vi "_PT_2DMCT_Example.vi"() -> ()   [LabVIEW 2026]
panel:
  out "ExtChData":dbl[][](array[numeric])
  in  "Timeout":i32
  in  "ExChs":i32
  in  "Frames":i32=1
  in  "Acq Trigger?":bool
  in  "Offset":i32=128 min=0 max=255 step=1
  out "Actual (us)":dbl
  in  "IntegrationTime (us)":dbl=0.1 min=0.1 max=5000.0 step=0.1
  out "MaxFrameRate":dbl
  in  "Frame Size (Row x Col)":u16(ring) items=["128x128", "96x128", "64x128", "32x128"]
  out "TempK":dbl
  out "First Image":dbl[][](graph)
  out "error":errorcluster
  # "INPUTS"
  # "OUTPUTS"
  # "Get Temp:"
  # "Set Frame Size:\n(optional)"
  # "Set Integration Time:"
  # "Set Offset:"
  # "Get Frames:"
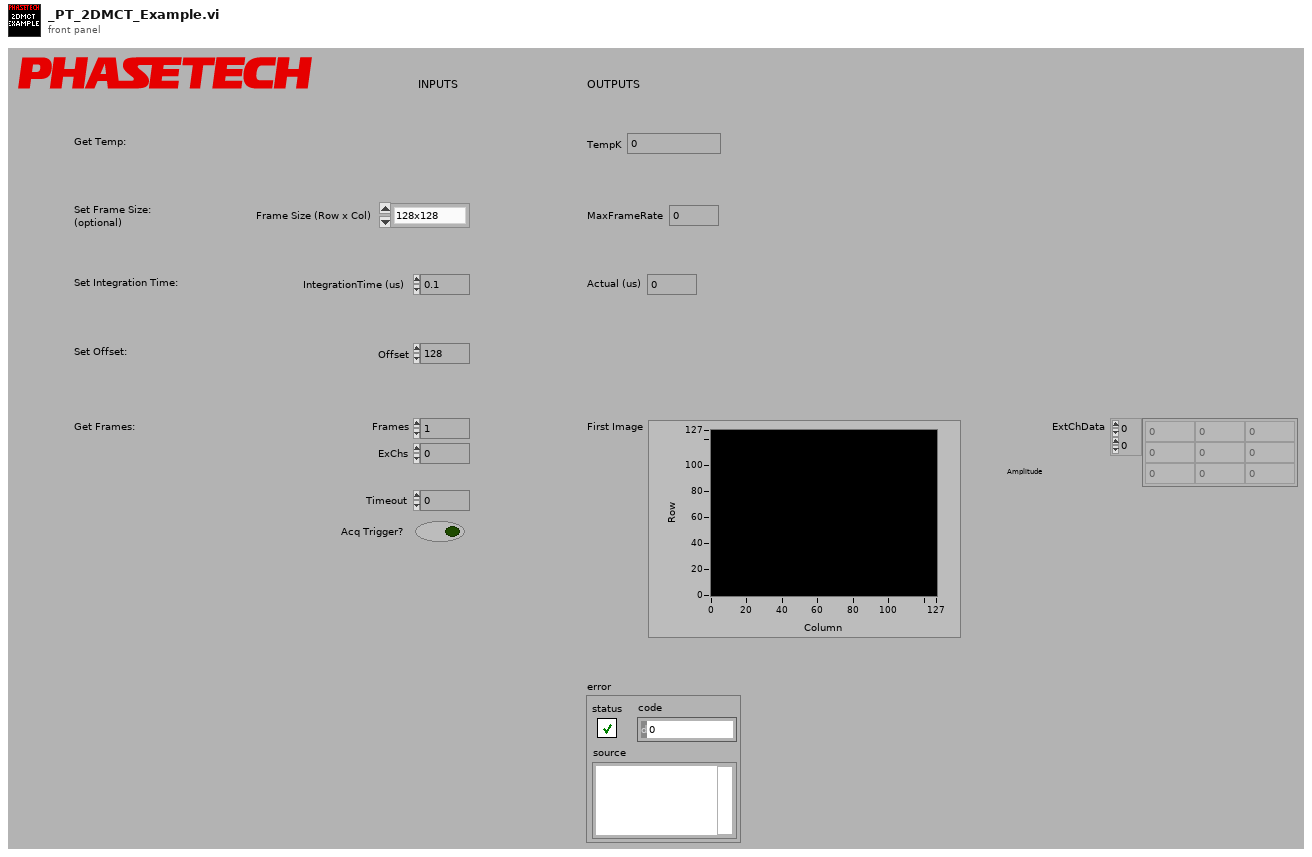
[diagram p1: front panel]
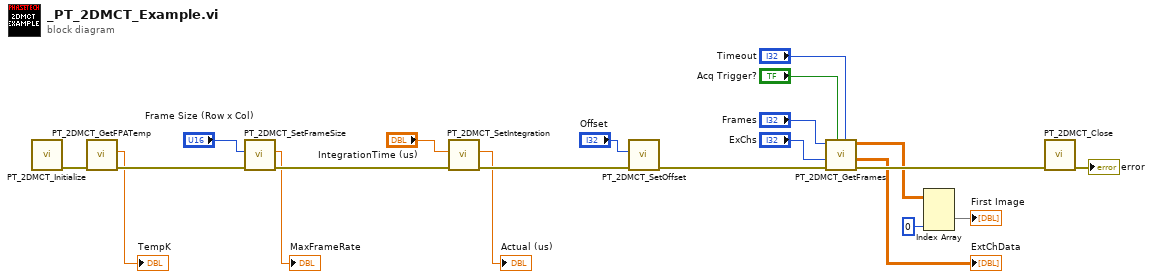
[diagram p0: block diagram]
diagram:
  n1 = call "PT_2DMCT_Initialize.vi"() -> ("error out"=w16:errorcluster)  [unwired: 11 in]
  n2 = call "PT_2DMCT_GetFPATemp.vi"("error in (no error)"=w16) -> ("error out"=w15:errorcluster, "TempK"=→"TempK":dbl)  [unwired: 8 in, 1 out]
  n3 = call "PT_2DMCT_SetFrameSize.vi"("error in (no error)"=w15, "Frame Size (Row x Col)"="Frame Size (Row x Col)") -> ("error out"=w14:errorcluster, "MaxFrameRate"=→"MaxFrameRate":dbl)  [unwired: 4 in]
  n4 = call "PT_2DMCT_SetIntegration.vi"("error in (no error)"=w14, "IntegrationTime (us)"="IntegrationTime (us)") -> ("error out"=w13:errorcluster, "Actual (us)"=→"Actual (us)":dbl)  [unwired: 4 in]
  n5 = call "PT_2DMCT_SetOffset.vi"("error in (no error)"=w13, "Offset"="Offset") -> ("error out"=w12:errorcluster)  [unwired: 9 in]
  n6 = call "PT_2DMCT_GetFrames.vi"("Timeout"="Timeout", "Acq Trigger?"="Acq Trigger?", "error in (no error)"=w12, "ExChs"="ExChs", "Frames"="Frames") -> ("error out"=w19:errorcluster, "ExtChData"=→"ExtChData":dbl[][], "FrameData"=w17:dbl[][][])  [unwired: 4 in]
  n7 = Index Array(array=w17, index (dim 2)=0 ("disabled index (col)")) -> (element=→"First Image":dbl[][])  [unwired: 2 in]
  n8 = call "PT_2DMCT_Close.vi"("error in (no error)"=w19) -> ("error out"=→"error":errorcluster)  [unwired: 10 in]
